vi "Create.vi"(8 "error in (no error)":errorcluster, 10 "Input":string) -> (0 "error out":errorcluster, 3 "Proto":refnum<class "Proto.lvclass">)   [LabVIEW 2021, in "Proto.lvclass"]
uses:
  Proto.lvclass
  Proto.lvclass/Proto.ctl
  Helpers/Helpers.lvlib
panel:
  out "Map":string[][](array[string])
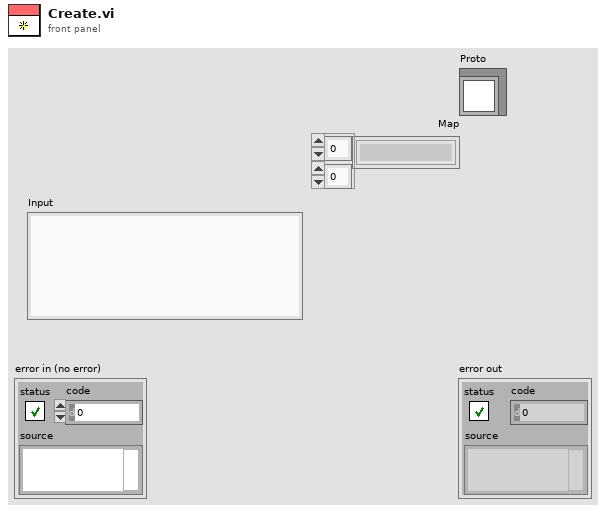
[diagram p1: front panel]
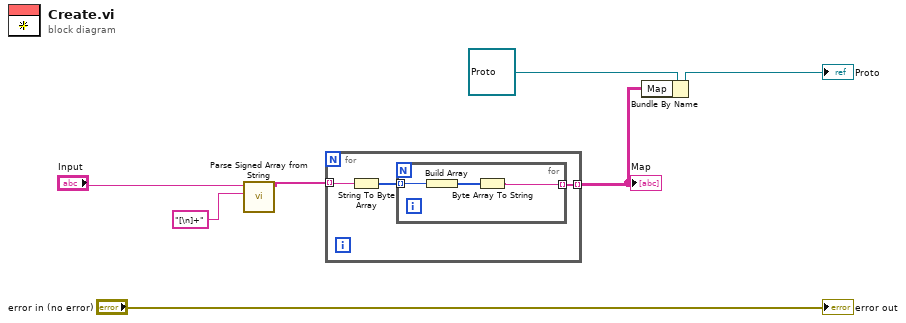
[diagram p0: block diagram]
diagram:
  n1 = call "Parse Signed Array from String.vi"("Delimiter regex"="[\n]+", "Input"="Input") -> ("Parsed Array"=w3:string[])  [unwired: 8 in, 1 out]
  n2 = for {
    tunnel: w3 -> [w10] mode=indexing
    tunnel: [w8] -> w1 mode=indexing
    n3 = String To Byte Array(string=w10) -> (unsigned byte array=w9:u8[])
    n4 = for {
      tunnel: w9 -> [w13] mode=indexing
      tunnel: [w11] -> w8 mode=indexing
      n5 = Build Array(w13) -> (w12:u8[])
      n6 = Byte Array To String(unsigned byte array=w12) -> (string=w11:string)
    }
  }
  "Map" <- w1
  n7 = Bundle By Name(cluster=refnum<class "Proto.lvclass"> refnum ("Proto"), "Map"=w1) -> (→"Proto":refnum<class "Proto.lvclass">)
  "error out" <- "error in (no error)"
